vi "MRC IMU Get Quaternion.vi"(8 "error in (no error)":errorcluster) -> (0 "error out":errorcluster, 3 "quaternion out":T1)   [LabVIEW 2026, in "MrcLib.lvlib"]
doc: "MRC_Status MRC_CALLCONV MRC_IMU_GetQuaternion(struct MRC_Quaternion* quaternion);"
uses:
  MrcLib.lvlib
  Types/MRC Quaternion.ctl
  MrcLib.dll
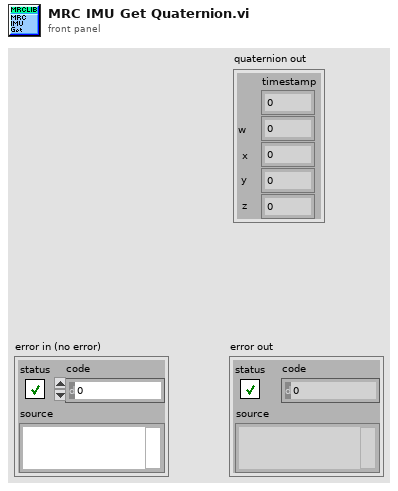
[diagram p1: front panel]
types:
  T1 = typedef "MrcLib.lvlib/MRC Quaternion.ctl" = cluster{"timestamp":i64, "w":dbl, "x":dbl, "y":dbl, "z":dbl}
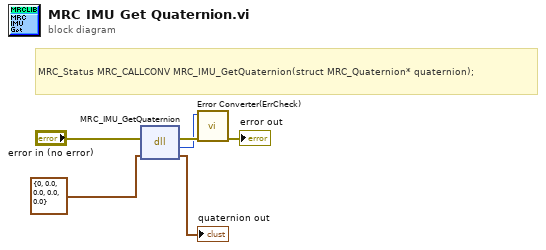
[diagram p0: block diagram]
diagram:
  # "MRC_Status MRC_CALLCONV MRC_IMU_GetQuaternion(struct MRC_Quaternion* quaternion);"
  n1 = dll-call lib="MrcLib.*" fn="MRC_IMU_GetQuaternion"(error in="error in (no error)", "quaternion"=T1 {"timestamp"=0, "w"=0.0, "x"=0.0, "y"=0.0, "z"=0.0}) -> (error out=w3:errorcluster, w1:i32, "quaternion"=→"quaternion out":T1)  [unwired: 2 in, 1 out]
  n2 = call "Error Converter(ErrCheck).vi"("error in (no error)"=w3, "status"=w1) -> ("error out"=→"error out":errorcluster)  [unwired: 9 in]
